vi "GetType.vi"(8 "error in (no error)":errorcluster, 11 "Configure Auto Zero Mode [AZ] Msg":refnum<class "Configure Auto Zero Mode [AZ] Msg.lvclass">) -> (0 "error out":errorcluster, 2 "Data Sample":variant, 3 "Configure Auto Zero Mode [AZ] Msg":refnum<class "Configure Auto Zero Mode [AZ] Msg.lvclass">)   [LabVIEW 2016, in "CS++DMM.lvlib" / "Configure Auto Zero Mode [AZ] Msg.lvclass"]
uses:
  Configure Auto Zero Mode [AZ] Msg.lvclass
  Configure Auto Zero Mode [AZ] Msg.lvclass/Configure Auto Zero Mode [AZ] Msg.ctl
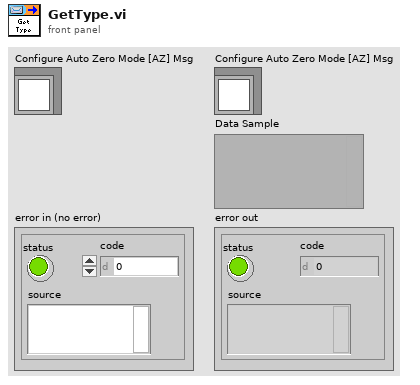
[diagram p1: front panel]
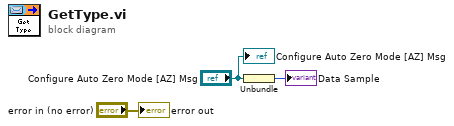
[diagram p0: block diagram]
diagram:
  n1 = Unbundle("Configure Auto Zero Mode [AZ] Msg") -> (→"Data Sample":i32)
  "error out" <- "error in (no error)"
  "Configure Auto Zero Mode [AZ] Msg" <- "Configure Auto Zero Mode [AZ] Msg"
